vi "Wrfm Info to Scales.vi"(11 "wfm info":T1(array[cluster])) -> (1 "Scaling coefficients":dbl[][](array[numeric]), 2 "dt":dbl, 3 "t0":dbl)   [LabVIEW 2016]
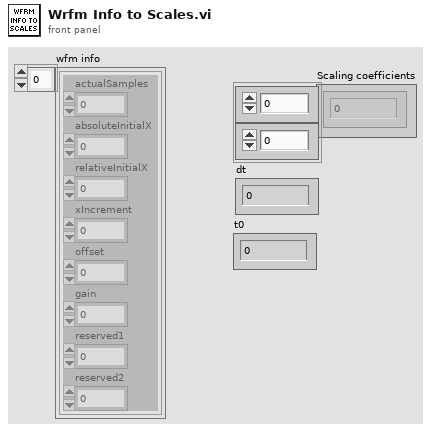
[diagram p1: front panel]
types:
  T1 = cluster{"actualSamples":i32, "absoluteInitialX":dbl, "relativeInitialX":dbl, "xIncrement":dbl, "offset":dbl, "gain":dbl, "reserved1":dbl, "reserved2":dbl}[]
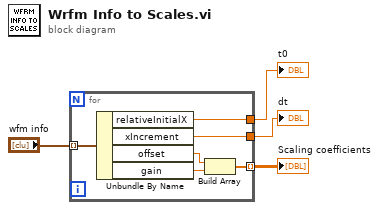
[diagram p0: block diagram]
diagram:
  n1 = for {
    tunnel: "wfm info" -> [w10] mode=indexing
    tunnel: [w9] -> w1
    tunnel: [w8] -> w2
    tunnel: [w5] -> w3 mode=indexing
    n2 = Unbundle By Name(w10) -> ("relativeInitialX"=w9:dbl, "xIncrement"=w8:dbl, "offset"=w7:dbl, "gain"=w6:dbl)
    n3 = Build Array(w7, w6) -> (w5:dbl[])
  }
  "Scaling coefficients" <- w3
  "dt" <- w2
  "t0" <- w1
